vi "pH Meter.vi"(11 "pH index":i32) -> ()   [LabVIEW 2015]
uses:
  gran.ctl
  save gran.ctl
  pH titration.ctl
  pH gran type.ctl
  pH Gran plot.ctl
  DAQ configuration/scale type.ctl
  DAQ configuration/Sensor buffer command.ctl
  Process Controller 3.0/Calibration and Function folders.ctl
panel:
  in  "Data interval (s)":ext=1.0 format="%.3f"
  in  "End Titration":bool
  in  "change Va":bool
  out "incremental titrant added":dbl format="%.3f"
  out "Gran Plot":T1={"Ve"=0.5, "ANC"=0.5, "r"=0.5, "Gran type"=enum."ANC", "Gran Plot"=[], "pH"=[]} {"r" format="%.4f"; "ANC" format="%.2p"; "Ve" format="%.3f"; "pH" format="%.2f"}
  in  "accept pH value":bool
  out "Titrating":bool
  out "Titration":T3 {"Nt" format="%.4f"; "Vo" format="%.3f"}
  in  "Save Gran Plot":T4
  in  "Create Gran Plot":T5
  in  "Default Buffers":T6(array[cluster])=[{"Buffer"=4.0, "Calibrated"=FALSE, "V/T"=0.0013599919516459151}, {"Buffer"=7.0, "Calibrated"=FALSE, "V/T"=0.0}, {"Buffer"=10.0, "Calibrated"=FALSE, "V/T"=0.0}] {"V/T" format="%.2f"; "Buffer" format="%.2f"}
  out "name":string
  out "units":string
  in  "Temperature\nChannel":i32 min=0 step=1
  in  "Temperature":dbl[unit]=273.15 format="%.1f"
  in  "Temperature\ncompensated":bool
  out "XY Graph":cluster{dbl[], dbl[]}[](graph)
  in  "OK Button":bool
  in  "add buffer smooth interval (s)":sgl=1.0 format="%.3f"
  in  "Clear buffers":bool
  in  "Edit buffers":bool
  in  "Add buffer":bool
  out "Quit":bool
  out "Buffers":T6(array[cluster]) {"V/T" format="%.2f"; "Buffer" format="%.2f"}
  out "Sample Temperature":dbl[unit] format="%.2f"
  out "pH":dbl format="%.3f"
  out "pH voltage":sgl[unit] format="%.1f"
  # "mL"
  # "eq/L"
  # "Normality of titrant"
  # "eq/L"
  # "mL"
  # "Volume of sample"
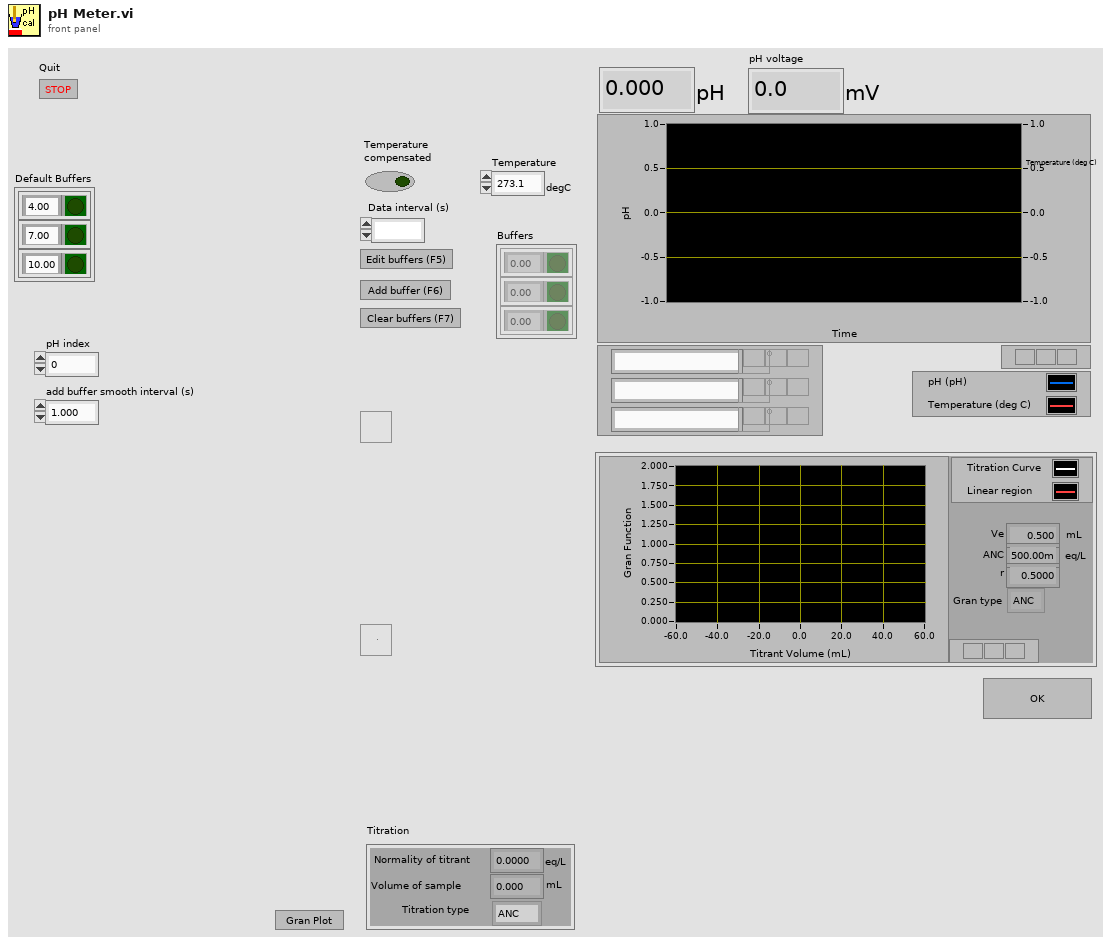
[diagram p1: front panel]
types:
  T1 = typedef "pH Gran plot.ctl" = cluster{"Ve":dbl, "ANC":dbl, "r":dbl, "Gran type":T2, "Gran Plot":cluster{"Va":dbl[], "F1":dbl[]}[], "pH":dbl[]}
  T2 = typedef "pH gran type.ctl" = enum16{"ANC", "BNC"}
  T3 = typedef "pH titration.ctl" = cluster{"Vo":dbl, "Nt":dbl, "Titration type":T2}
  T4 = typedef "save gran.ctl" = bool
  T5 = typedef "gran.ctl" = bool
  T6 = cluster{"Buffer":dbl, "Calibrated":bool, "V/T":dbl}[]
  T7 = typedef "Sensor buffer command.ctl" = enum16{"read average", "read recent", "read all", "write", "set buffer size", "Read channel config", "Write channel config", "clear"}
  T8 = typedef "scale type.ctl" = enum16{"Volts", "Polynomial", "Correspondence Table", "pH", "Dissolved Oxygen", "Quadratic", "Photometer"}
  T9 = typedef "Calibration and Function folders.ctl" = enum16{"Sensors", "Functions", "Config File", "PublicAppFolder", "New ini File", "Set Config File", "Delete ini File"}
  T10 = typedef "Channel config.ctl" = cluster{"Channel Indices":T11[], "AI Max voltage":dbl[], "Calibration matrix":T12}
  T11 = typedef "channel identifier.ctl" = u16
  T12 = typedef "calib array.ctl" = T13[]
  T13 = typedef "conversion.ctl" = cluster{"conversion matrix":sgl[][], "units":string, "name":string, "scale type":T8, "offset (volts)":dbl, "second channel":i8, "correspondence table":T14, "offset (physical units)":dbl, "pH scale":T15, "D.O.":T16, "Photometer data":T17}
  T14 = typedef "correspondence table.ctl" = cluster{"physical units":dbl, "volts":dbl}[]
  T15 = typedef "pH scale.ctl" = cluster{"Buffers":cluster{"Buffer":dbl, "Calibrated":bool, "V/T":dbl}[], "Temperature":dbl}
  T16 = typedef "DO scale.ctl" = cluster{"Temperature":dbl, "K":dbl, "barometric pressure":dbl}
  T17 = typedef "Photometer calibration data.ctl" = cluster{"Dark Voltage":dbl, "Blank Voltage":dbl, "Standards":cluster{"Concentration":dbl, "Voltage":dbl}[]}
  T18 = cluster{"Buffer":dbl, "Calibrated":bool, "V/T":dbl}
  T19 = typedef "Sensor data.ctl" = cluster{" Sensor array":T20[], "Time":dbl}
  T20 = typedef "sensor cluster.ctl" = cluster{"voltage":sgl, "scaled":sgl, "units":string, "Out of Range":bool}
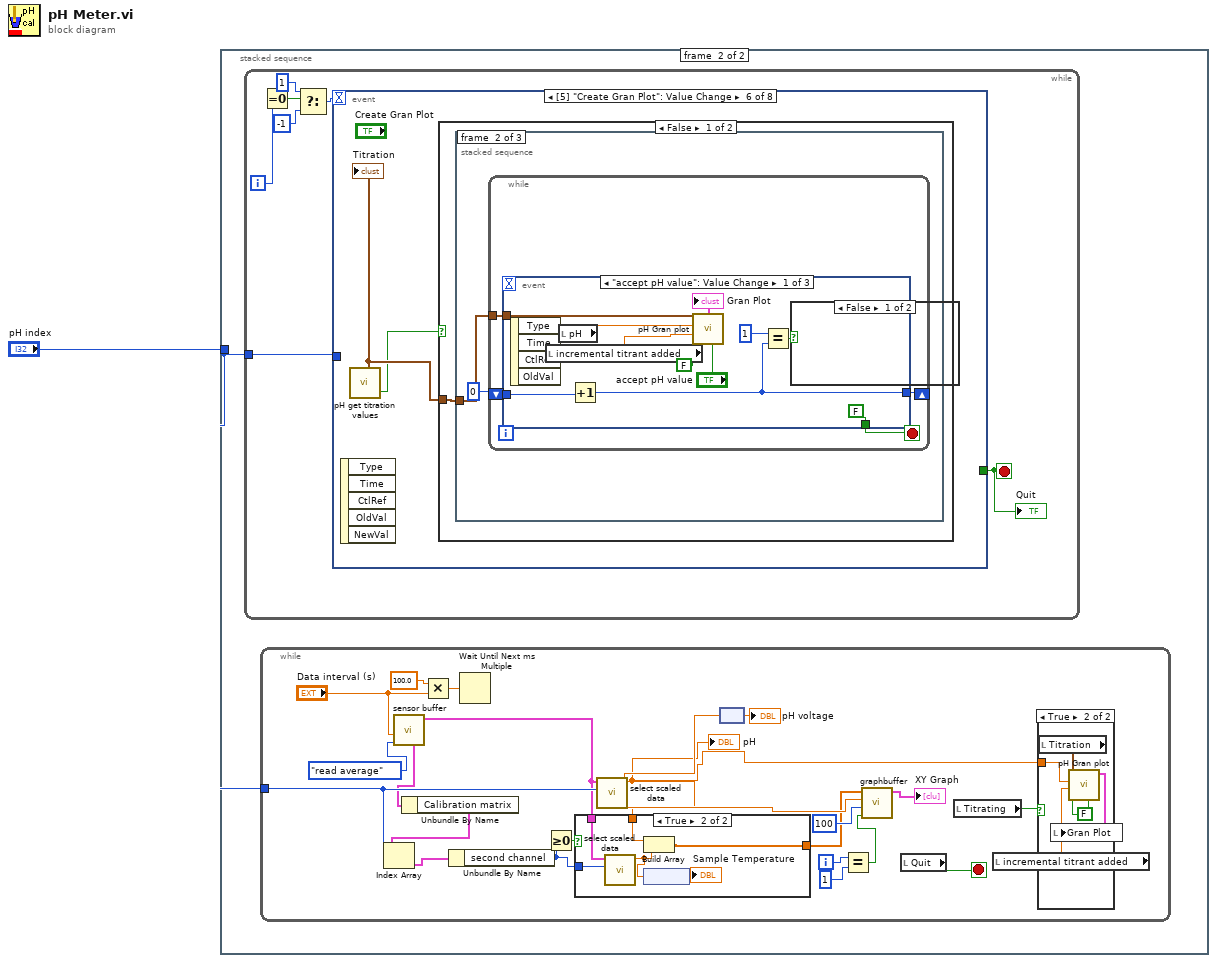
[diagram p0: block diagram]
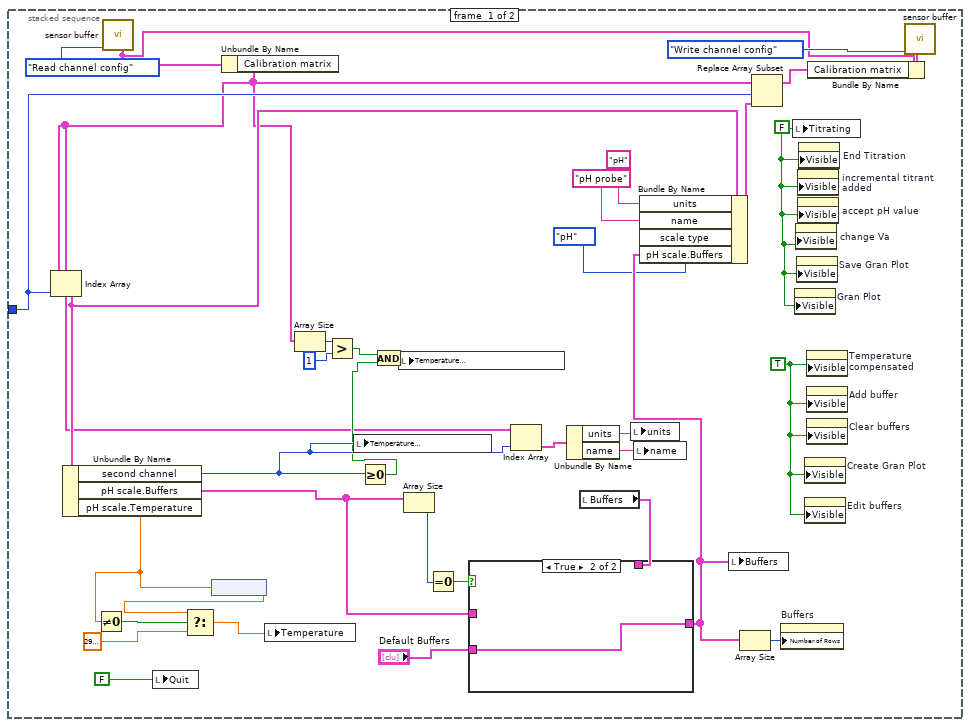
[diagram p2: hidden frame]
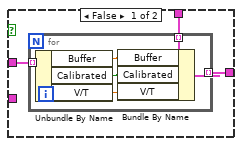
[diagram p3: hidden frame]
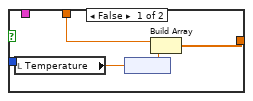
[diagram p5: hidden frame]
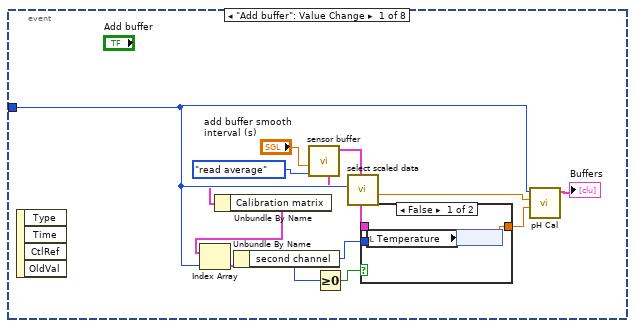
[diagram p6: hidden frame]
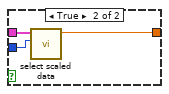
[diagram p7: hidden frame]
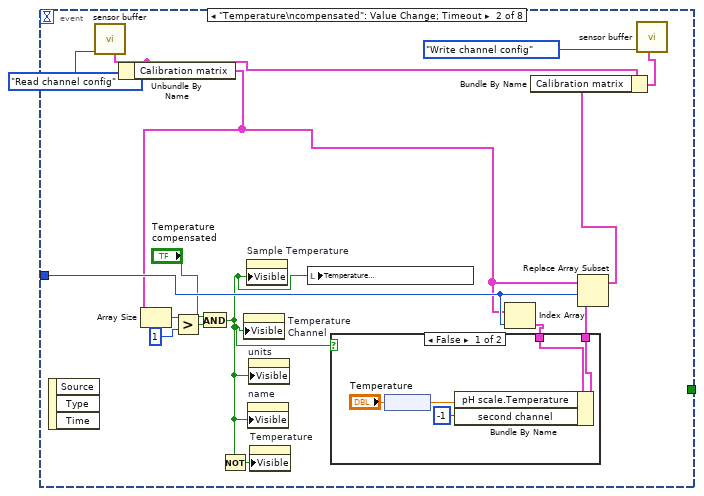
[diagram p8: hidden frame]
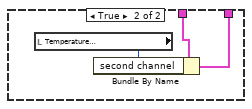
[diagram p9: hidden frame]
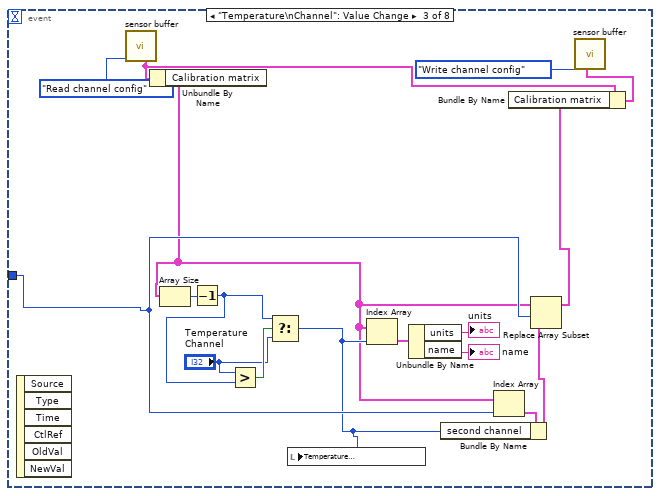
[diagram p10: hidden frame]
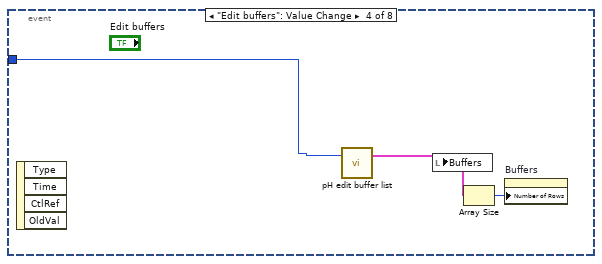
[diagram p11: hidden frame]
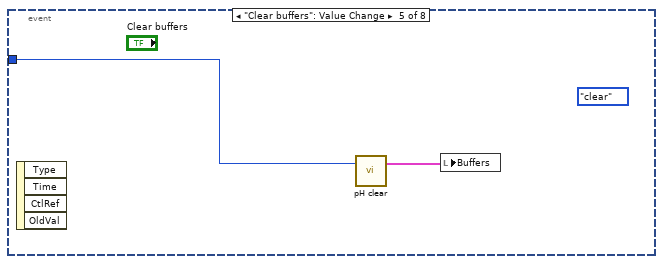
[diagram p12: hidden frame]
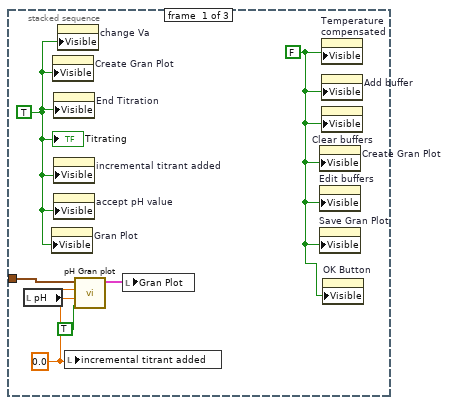
[diagram p13: hidden frame]
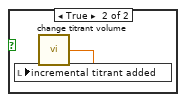
[diagram p14: hidden frame]
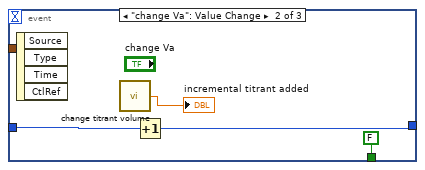
[diagram p15: hidden frame]
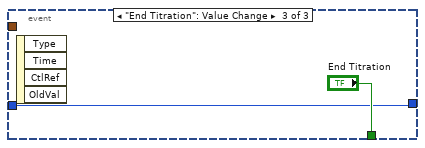
[diagram p16: hidden frame]
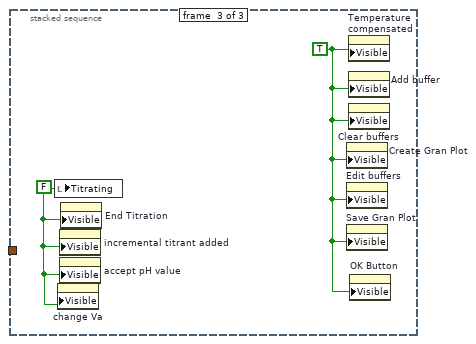
[diagram p17: hidden frame]
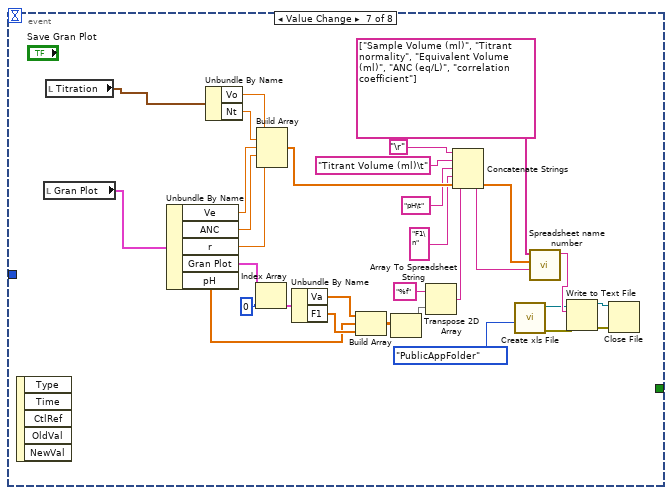
[diagram p19: hidden frame]
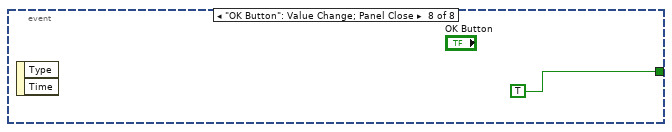
[diagram p20: hidden frame]
diagram:
  n1 = stacked-sequence {
    tunnel: "pH index" -> [w28 w48]
    frame #0 {
      w4 = TRUE ("Visible")
      w3 = FALSE ("Visible")
      n2 = call "sensor buffer.vi"("command"=Sensor_buffer_command."Read channel config") -> ("Channel Config out"=w9:T10)  [unwired: 6 in, 4 out]
      n3 = local write "Quit"(FALSE ("Quit")) -> ()
      n4 = Unbundle By Name(w9) -> ("Calibration matrix"=w11:T12)
      n5 = Index Array(array=w11, index=w28) -> (element=w27:T13)
      n6 = Unbundle By Name(w27) -> ("second channel"=w35:i8, "pH scale.Buffers"=w31:T6, "pH scale.Temperature"=w18:dbl)
      n7 = Not Equal To 0?(x=w18) -> (x != 0?=w17:bool)
      n8 = node(w18) -> (w16:dbl[unit])
      n9 = Select(t=w16, s=w17, f=dbl[unit] 295.15) -> (s? t:f=w15:dbl[unit])
      n10 = local write "Temperature"(w15) -> ()
      n11 = Array Size(array=w11) -> (size(s)=w23:i32)
      n12 = Greater?(x=w23, y=1) -> (0:w21:bool)
      n13 = local write "Temperature\nChannel"(w35) -> ()
      n14 = Greater Or Equal To 0?(x=w35) -> (x >= 0?=w20:bool)
      n15 = And(x=w21, y=w20) -> (x .and. y?=w19:bool)
      n16 = local write "Temperature\ncompensated"(w19) -> ()
      n17 = Array Size(array=w31) -> (size(s)=w29:i32)
      n18 = Equal To 0?(x=w29) -> (x = 0?=w30:bool)
      n19 = Index Array(array=w11, index=w35) -> (element=w34:T13)
      n20 = Unbundle By Name(w34) -> ("units"=w33:string, "name"=w32:string)
      n21 = local read "Buffers"() -> (w36:T6)
      n22 = case shown="True" w30 {
        tunnel: w31 -> [w40 _]
        tunnel: w36 -> [w39 _]
        tunnel: [w38 w47] -> w24
        tunnel: "Default Buffers" -> [_ w47]
        frame False {
          n23 = for {
            tunnel: w40 -> [w46] mode=indexing
            tunnel: w39 -> [w45] mode=indexing
            tunnel: [w42] -> w38 mode=indexing
            n24 = Unbundle By Name(w46) -> ("Buffer"=w44:dbl, "Calibrated"=w43:bool, "V/T"=w41:dbl)
            n25 = Bundle By Name(cluster=w45, "Buffer"=w44, "Calibrated"=w43, "V/T"=w41) -> (w42:T18)
          }
        }
        frame True {
        }
      }
      n26 = local write "units"(w33) -> ()
      n27 = local write "name"(w32) -> ()
      n28 = Bundle By Name(cluster=w27, "units"="pH", "name"="pH probe", "scale type"=scale_type."pH", "pH scale.Buffers"=w24) -> (w26:T13)
      n29 = local write "Buffers"(w24) -> ()
      n30 = Array Size(array=w24) -> (size(s)=w37:i32)
      n31 = Replace Array Subset(array=w11, new element=w26, index=w28) -> (w8:T12)
      n32 = property on="Buffers" class="Arr (strict)"("Number of Rows"=w37) -> ()  [unwired: 2 in, 2 out]
      n33 = local write "Titrating"(w3) -> ()
      n34 = property on="Gran Plot" class="Clust (strict)"("Visible"=w3) -> ()  [unwired: 2 in, 2 out]
      n35 = property on="change Va" class="Bool"("Visible"=w3) -> ()  [unwired: 2 in, 2 out]
      n36 = property on="Save Gran Plot" class="Bool"("Visible"=w3) -> ()  [unwired: 2 in, 2 out]
      n37 = property on="incremental titrant added" class="DigNum (strict)"("Visible"=w3) -> ()  [unwired: 2 in, 2 out]
      n38 = property on="accept pH value" class="Bool"("Visible"=w3) -> ()  [unwired: 2 in, 2 out]
      n39 = property on="End Titration" class="Bool"("Visible"=w3) -> ()  [unwired: 2 in, 2 out]
      n40 = property on="Create Gran Plot" class="Bool"("Visible"=w4) -> ()  [unwired: 2 in, 2 out]
      n41 = property on="Edit buffers" class="Bool"("Visible"=w4) -> ()  [unwired: 2 in, 2 out]
      n42 = property on="Temperature\ncompensated" class="Bool (strict)"("Visible"=w4) -> ()  [unwired: 2 in, 2 out]
      n43 = property on="Add buffer" class="Bool"("Visible"=w4) -> ()  [unwired: 2 in, 2 out]
      n44 = property on="Clear buffers" class="Bool"("Visible"=w4) -> ()  [unwired: 2 in, 2 out]
      n45 = Bundle By Name(cluster=w9, "Calibration matrix"=w8) -> (w7:T10)
      n46 = call "sensor buffer.vi"("Channel Config"=w7, "command"=Sensor_buffer_command."Write channel config") -> ()  [unwired: 5 in, 5 out]
    }
    frame #1 {
      n47 = while {
        tunnel: w48 -> [w92]
        i -> [w88]
        stop <- w93 stop-if-true
        n48 = Equal To 0?(x=w88) -> (x = 0?=w87:bool)
        n49 = Select(t=1, s=w87, f=-1) -> (s? t:f=w89:i32)
        n50 = event shown="[5] \"Create Gran Plot\": Value Change" {
          selector: _ -> [_ _ _ _ _ _ _ _]
          dyn-events: _ -> [_ _ _ _ _ _ _ _]
          timeout: w89 -> [_ _ _ _ _ _ _ _]
          tunnel: [_ _ _ _ _ _ _ TRUE ("OK Button")] -> w93
          tunnel: w92 -> [w105 w122 w147 w151 w154 _ _ _]
          event "Add buffer": Value Change {
            n51 = event-data() -> ()  [unwired: 1 in, 4 out]
            n52 = call "sensor buffer.vi"("command"=Sensor_buffer_command."read average", "smooth interval (s)"="add buffer smooth interval (s)") -> ("Calibrated data"=w96:T19, "Channel Config out"=w95:T10)  [unwired: 5 in, 3 out]
            n53 = Unbundle By Name(w95) -> ("Calibration matrix"=w94:T12)
            n54 = Index Array(array=w94, index=w105) -> (element=w101:T13)
            n55 = Unbundle By Name(w101) -> ("second channel"=w100:i8)
            n56 = Greater Or Equal To 0?(x=w100) -> (x >= 0?=w99:bool)
            n57 = call "select scaled data.vi"("Sensor index"=w105, "Sensor Data"=w96) -> ("voltage"=w104:sgl)  [unwired: 4 in, 5 out]
            n58 = case shown="False" w99 {
              tunnel: w96 -> [_ w110]
              tunnel: [w106 w109] -> w103
              tunnel: w100 -> [_ w108]
              frame False {
                n59 = local read "Temperature"() -> (w107:dbl[unit])
                n60 = node(w107) -> (w106:dbl)
              }
              frame True {
                n61 = call "select scaled data.vi"("Sensor index"=w108, "Sensor Data"=w110) -> ("scaled"=w109:sgl)  [unwired: 4 in, 5 out]
              }
            }
            n62 = call "pH Cal.vi"("index"=w105, "pH voltage"=w104, "Temperature"=w103) -> ("Buffers"=→"Buffers":T6)  [unwired: 7 in]
          }
          event "Temperature\ncompensated": Value Change; Timeout {
            n63 = event-data() -> ()  [unwired: 1 in, 3 out]
            n64 = call "sensor buffer.vi"("command"=Sensor_buffer_command."Read channel config") -> ("Channel Config out"=w113:T10)  [unwired: 6 in, 4 out]
            n65 = Unbundle By Name(w113) -> ("Calibration matrix"=w115:T12)
            n66 = Array Size(array=w115) -> (size(s)=w121:i32)
            n67 = Greater?(x=w121, y=1) -> (0:w119:bool)
            n68 = And(x="Temperature\ncompensated", y=w119) -> (x .and. y?=w117:bool)
            n69 = Not(x=w117) -> (.not. x?=w125:bool)
            n70 = property on="Temperature\nChannel" class="DigNum (strict)"("Visible"=w117) -> ()  [unwired: 2 in, 2 out]
            n71 = property on="Sample Temperature" class="DigNum (strict)"("Visible"=w117) -> ()  [unwired: 2 in, 2 out]
            n72 = property on="name" class="Str"("Visible"=w117) -> ()  [unwired: 2 in, 2 out]
            n73 = property on="units" class="Str"("Visible"=w117) -> ()  [unwired: 2 in, 2 out]
            n74 = property on="Temperature" class="DigNum (strict)"("Visible"=w125) -> ()  [unwired: 2 in, 2 out]
            n75 = local write "Temperature\ncompensated"(w117) -> ()
            n76 = Index Array(array=w115, index=w122) -> (element=w124:T13)
            n77 = case shown="False" w117 {
              tunnel: w124 -> [w130 w132]
              tunnel: [w129 w131] -> w123
              frame False {
                n78 = node("Temperature") -> (w127:dbl)
                n79 = Bundle By Name(cluster=w130, "pH scale.Temperature"=w127, "second channel"=i8 -1) -> (w129:T13)
              }
              frame True {
                n80 = local read "Temperature\nChannel"() -> (w133:i32)
                n81 = Bundle By Name(cluster=w132, "second channel"=w133) -> (w131:T13)
              }
            }
            n82 = Replace Array Subset(array=w115, new element=w123, index=w122) -> (w112:T12)
            n83 = Bundle By Name(cluster=w113, "Calibration matrix"=w112) -> (w111:T10)
            n84 = call "sensor buffer.vi"("Channel Config"=w111, "command"=Sensor_buffer_command."Write channel config") -> ()  [unwired: 5 in, 5 out]
          }
          event "Temperature\nChannel": Value Change {
            n85 = event-data() -> ()  [unwired: 1 in, 6 out]
            n86 = call "sensor buffer.vi"("command"=Sensor_buffer_command."Read channel config") -> ("Channel Config out"=w136:T10)  [unwired: 6 in, 4 out]
            n87 = Unbundle By Name(w136) -> ("Calibration matrix"=w138:T12)
            n88 = Array Size(array=w138) -> (size(s)=w144:i32)
            n89 = Decrement(x=w144) -> (x-1=w142:i32)
            n90 = Greater?(x="Temperature\nChannel", y=w142) -> (0:w143:bool)
            n91 = Select(t=w142, s=w143, f="Temperature\nChannel") -> (s? t:f=w140:i32)
            n92 = local write "Temperature\nChannel"(w140) -> ()
            n93 = Index Array(array=w138, index=w140) -> (element=w150:T13)
            n94 = Unbundle By Name(w150) -> ("units"=→"units":string, "name"=→"name":string)
            n95 = Index Array(array=w138, index=w147) -> (element=w145:T13)
            n96 = Bundle By Name(cluster=w145, "second channel"=w140) -> (w146:T13)
            n97 = Replace Array Subset(array=w138, new element=w146, index=w147) -> (w135:T12)
            n98 = Bundle By Name(cluster=w136, "Calibration matrix"=w135) -> (w134:T10)
            n99 = call "sensor buffer.vi"("Channel Config"=w134, "command"=Sensor_buffer_command."Write channel config") -> ()  [unwired: 5 in, 5 out]
          }
          event "Edit buffers": Value Change {
            n100 = event-data() -> ()  [unwired: 1 in, 4 out]
            n101 = call "pH edit buffer list.vi"("index"=w151) -> ("Buffers out"=w152:T6)  [unwired: 2 in]
            n102 = local write "Buffers"(w152) -> ()
            n103 = Array Size(array=w152) -> (size(s)=w153:i32)
            n104 = property on="Buffers" class="Arr (strict)"("Number of Rows"=w153) -> ()  [unwired: 2 in, 2 out]
          }
          event "Clear buffers": Value Change {
            (unwired) Sensor_buffer_command."clear" ("command")
            n105 = event-data() -> ()  [unwired: 1 in, 4 out]
            n106 = call "pH clear.vi"("index"=w154) -> ("Buffers"=w155:T6)  [unwired: 2 in]
            n107 = local write "Buffers"(w155) -> ()
          }
          event Value Change {
            n108 = event-data() -> ()  [unwired: 1 in, 5 out]
            n109 = call "pH get titration values.vi"() -> ("canceled"=w156:bool, "Titration"=w157:T3)  [unwired: 2 in]
            "Titration" <- w157
            n110 = case shown="False" w156 {
              tunnel: w157 -> [w158 _]
              frame False {
                n111 = stacked-sequence {
                  tunnel: w158 -> [w163 w167 _]
                  frame #0 {
                    w159 = FALSE ("Visible")
                    w162 = 0.0 ("incremental titrant added")
                    w160 = TRUE ("Visible")
                    n112 = local read "pH"() -> (w165:dbl)
                    n113 = property on="Gran Plot" class="Clust (strict)"("Visible"=w160) -> ()  [unwired: 2 in, 2 out]
                    n114 = property on="Create Gran Plot" class="Bool"("Visible"=w160) -> ()  [unwired: 2 in, 2 out]
                    n115 = property on="End Titration" class="Bool"("Visible"=w160) -> ()  [unwired: 2 in, 2 out]
                    n116 = property on="incremental titrant added" class="DigNum (strict)"("Visible"=w160) -> ()  [unwired: 2 in, 2 out]
                    n117 = property on="accept pH value" class="Bool"("Visible"=w160) -> ()  [unwired: 2 in, 2 out]
                    n118 = property on="change Va" class="Bool"("Visible"=w160) -> ()  [unwired: 2 in, 2 out]
                    n119 = local write "incremental titrant added"(w162) -> ()
                    n120 = call "pH Gran plot.vi"("initialize"=TRUE, "amount of titrant added"=w162, "pH"=w165, "sample"=w163) -> ("Gran plot"=w161:T1)  [unwired: 7 in]
                    n121 = local write "Gran Plot"(w161) -> ()
                    n122 = property on="Create Gran Plot" class="Bool"("Visible"=w159) -> ()  [unwired: 2 in, 2 out]
                    n123 = property on="Edit buffers" class="Bool"("Visible"=w159) -> ()  [unwired: 2 in, 2 out]
                    n124 = property on="Save Gran Plot" class="Bool"("Visible"=w159) -> ()  [unwired: 2 in, 2 out]
                    n125 = property on="Temperature\ncompensated" class="Bool (strict)"("Visible"=w159) -> ()  [unwired: 2 in, 2 out]
                    n126 = property on="Add buffer" class="Bool"("Visible"=w159) -> ()  [unwired: 2 in, 2 out]
                    n127 = property on="Clear buffers" class="Bool"("Visible"=w159) -> ()  [unwired: 2 in, 2 out]
                    n128 = property on="OK Button" class="Bool"("Visible"=w159) -> ()  [unwired: 2 in, 2 out]
                    "Titrating" <- w160
                  }
                  frame #1 {
                    n129 = while {
                      tunnel: w167 -> [w170]
                      shift-right: [w168] -> _
                      shift-left: 0 -> [w169]
                      stop <- w171 stop-if-true
                      n130 = event shown="[0] \"accept pH value\": Value Change" {
                        selector: _ -> [_ _ _]
                        dyn-events: _ -> [_ _ _]
                        timeout: _ -> [_ _ _]
                        tunnel: [FALSE ("End Titration") FALSE ("End Titration") "End Titration"] -> w171
                        tunnel: w170 -> [w182 _ _]
                        tunnel: w169 -> [w175 w186 w188]
                        tunnel: [w173 w185 w188] -> w168
                        event "accept pH value": Value Change {
                          n131 = event-data() -> ()  [unwired: 1 in, 4 out]
                          n132 = local read "incremental titrant added"() -> (w176:dbl)
                          n133 = local read "pH"() -> (w181:dbl)
                          n134 = Increment(x=w175) -> (x+1=w173:i32)
                          n135 = call "pH Gran plot.vi"("accept pH value"="accept pH value", "initialize"=FALSE, "amount of titrant added"=w176, "pH"=w181, "sample"=w182) -> ("Gran plot"=→"Gran Plot":T1)  [unwired: 6 in]
                          n136 = Equal?(x=1, y=w173) -> (x = y?=w174:bool)
                          n137 = case shown="False" w174 {
                            frame False {
                            }
                            frame True {
                              n138 = call "change titrant volume.vi"() -> ("incremental titrant added out"=w183:dbl)  [unwired: 2 in]
                              n139 = local write "incremental titrant added"(w183) -> ()
                            }
                          }
                        }
                        event "change Va": Value Change {
                          n140 = event-data() -> ()  [unwired: 1 in, 4 out]
                          n141 = call "change titrant volume.vi"() -> ("incremental titrant added out"=→"incremental titrant added":dbl)  [unwired: 2 in]
                          n142 = Increment(x=w186) -> (x+1=w185:i32)
                        }
                        event "End Titration": Value Change {
                          n143 = event-data() -> ()  [unwired: 1 in, 4 out]
                        }
                      }
                    }
                  }
                  frame #2 {
                    w190 = TRUE ("Visible")
                    w191 = FALSE ("Visible")
                    n144 = local write "Titrating"(w191) -> ()
                    n145 = property on="change Va" class="Bool"("Visible"=w191) -> ()  [unwired: 2 in, 2 out]
                    n146 = property on="incremental titrant added" class="DigNum (strict)"("Visible"=w191) -> ()  [unwired: 2 in, 2 out]
                    n147 = property on="accept pH value" class="Bool"("Visible"=w191) -> ()  [unwired: 2 in, 2 out]
                    n148 = property on="End Titration" class="Bool"("Visible"=w191) -> ()  [unwired: 2 in, 2 out]
                    n149 = property on="Create Gran Plot" class="Bool"("Visible"=w190) -> ()  [unwired: 2 in, 2 out]
                    n150 = property on="Edit buffers" class="Bool"("Visible"=w190) -> ()  [unwired: 2 in, 2 out]
                    n151 = property on="Save Gran Plot" class="Bool"("Visible"=w190) -> ()  [unwired: 2 in, 2 out]
                    n152 = property on="Temperature\ncompensated" class="Bool (strict)"("Visible"=w190) -> ()  [unwired: 2 in, 2 out]
                    n153 = property on="Add buffer" class="Bool"("Visible"=w190) -> ()  [unwired: 2 in, 2 out]
                    n154 = property on="Clear buffers" class="Bool"("Visible"=w190) -> ()  [unwired: 2 in, 2 out]
                    n155 = property on="OK Button" class="Bool"("Visible"=w190) -> ()  [unwired: 2 in, 2 out]
                  }
                }
              }
              frame True {
              }
            }
          }
          event Value Change {
            n156 = event-data() -> ()  [unwired: 1 in, 5 out]
            n157 = local read "Gran Plot"() -> (w210:T1)
            n158 = local read "Titration"() -> (w211:T3)
            n159 = Unbundle By Name(w210) -> ("Ve"=w217:dbl, "ANC"=w218:dbl, "r"=w219:dbl, "Gran Plot"=w212:cluster{"Va":dbl[], "F1":dbl[]}[], "pH"=w215:dbl[])
            n160 = Unbundle By Name(w211) -> ("Vo"=w221:dbl, "Nt"=w220:dbl)
            n161 = Index Array(array=w212, index=0) -> (element=w214:cluster{"Va":dbl[], "F1":dbl[]})
            n162 = Build Array(w221, w220, w217, w218, w219) -> (w207:dbl[])
            n163 = Unbundle By Name(w214) -> ("Va"=w208:dbl[], "F1"=w216:dbl[])
            n164 = Build Array(w208, w215, w216) -> (w206:dbl[][])
            n165 = Transpose 2D Array(2D array=w206) -> (transposed array=w192:dbl[][])
            n166 = Array To Spreadsheet String(array=w192, 3:"%f" ("format string")) -> (spreadsheet string=w197:string)  [unwired: 1 in]
            n167 = Concatenate Strings("\r", "Titrant Volume (ml)\t", "pH\t", "F1\n", w197) -> (w198:string)
            n168 = call "Create xls File.vi"("Folder"=Calibration_and_Function_folders."PublicAppFolder") -> ("error out"=w204:errorcluster, "refnum"=w194:refnum<file>)  [unwired: 3 in, 2 out]
            n169 = call "Spreadsheet name number.vi"("Terminal String"=w198, "Numbers"=w207, "Names"=string[] ["Sample Volume (ml)", "Titrant normality", "Equivalent Volume (ml)", "ANC (eq/L)", "correlation coefficient"]) -> ("Spreadsheet String"=w203:string)  [unwired: 7 in, 1 out]
            n170 = Write to Text File(file (use dialog)=w194, text=w203, error in=w204) -> (refnum out=w202:refnum<file>, error out=w201:errorcluster)  [unwired: 1 in, 1 out]
            n171 = Close File(refnum=w202, error in=w201) -> ()  [unwired: 2 out]
          }
          event "OK Button": Value Change; Panel Close {
            n172 = event-data() -> ()  [unwired: 1 in, 2 out]
          }
        }
        "Quit" <- w93
      }
      n173 = while {
        tunnel: w48 -> [w62]
        i -> [w57]
        stop <- w71 stop-if-true
        n174 = call "sensor buffer.vi"("command"=Sensor_buffer_command."read average", "smooth interval (s)"="Data interval (s)") -> ("Calibrated data"=w54:T19, "Channel Config out"=w53:T10)  [unwired: 5 in, 3 out]
        n175 = Unbundle By Name(w53) -> ("Calibration matrix"=w52:T12)
        n176 = Index Array(array=w52, index=w62) -> (element=w63:T13)
        n177 = Multiply(x=100.0 ("y"), y="Data interval (s)") -> (x*y=w70:ext)
        n178 = Unbundle By Name(w63) -> ("second channel"=w60:i8)
        n179 = Wait Until Next ms Multiple(millisecond multiple=w70) -> ()  [unwired: 1 out]
        n180 = Greater Or Equal To 0?(x=w60) -> (x >= 0?=w59:bool)
        n181 = call "select scaled data.vi"("Sensor index"=w62, "Sensor Data"=w54) -> ("voltage"=w61:sgl, "scaled"=w50:sgl, "Time"=w68:dbl)  [unwired: 4 in, 3 out]
        "pH" <- w50
        n182 = case shown="True" w59 {
          tunnel: w54 -> [_ w86]
          tunnel: w60 -> [_ w85]
          tunnel: w50 -> [w80 w84]
          tunnel: [w79 w83] -> w58
          frame False {
            n183 = local read "Temperature"() -> (w78:dbl[unit])
            n184 = node(w78) -> (w77:dbl)
            n185 = Build Array(w80, w77) -> (w79:dbl[])
          }
          frame True {
            n186 = call "select scaled data.vi"("Sensor index"=w85, "Sensor Data"=w86) -> ("scaled"=w81:sgl)  [unwired: 4 in, 5 out]
            n187 = Build Array(w84, w81) -> (w83:sgl[])
            n188 = node(w81) -> (→"Sample Temperature":sgl[unit])
          }
        }
        n189 = node(w61) -> (→"pH voltage":sgl[unit])
        n190 = Equal?(x=w57, y=1) -> (x = y?=w66:bool)
        n191 = call "graphbuffer.vi"("Reset"=w66, "history length"=u16 100, "Time"=w68, "data"=w58) -> ("Multiplot graph data"=→"XY Graph":cluster{dbl[], dbl[]}[])  [unwired: 5 in, 2 out]
        n192 = local read "Quit"() -> (w71:bool)
        n193 = local read "Titrating"() -> (w51:bool)
        n194 = case shown="True" w51 {
          tunnel: w50 -> [_ w75]
          frame False {
          }
          frame True {
            w72 = FALSE ("accept pH value")
            n195 = local read "incremental titrant added"() -> (w74:dbl)
            n196 = local read "Titration"() -> (w76:T3)
            n197 = call "pH Gran plot.vi"("accept pH value"=w72, "initialize"=w72, "amount of titrant added"=w74, "pH"=w75, "sample"=w76) -> ("Gran plot"=w73:T1)  [unwired: 6 in]
            n198 = local write "Gran Plot"(w73) -> ()
          }
        }
      }
    }
  }
